vi "Triggers To Buttons.vi"(10 "Down":dbl, 11 "Up":dbl) -> (2 "Right":bool, 3 "Left":bool)   [LabVIEW 2014]
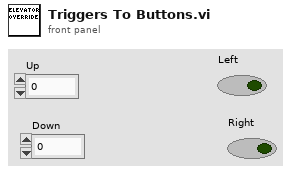
[diagram p1: front panel]
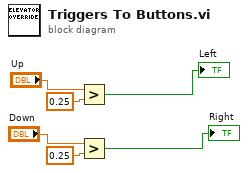
[diagram p0: block diagram]
diagram:
  n1 = Greater?(x="Up", y=0.25) -> (0:→"Left":bool)
  n2 = Greater?(x="Down", y=0.25) -> (0:→"Right":bool)
